vi "ZMQ subscriber example.vi"() -> ()   [LabVIEW 2018]
uses:
  <vilib>/addons/zeromq/socket_type.ctl
  <vilib>/addons/zeromq/socket_options.ctl
  <vilib>/addons/zeromq/zeromq.lvlib
  <vilib>/addons/zeromq/zmq_context.lvclass
  <vilib>/addons/zeromq/zmq_socket.lvclass
panel:
  in  "Display all data":bool
  out "error out":errorcluster
  out "data":string
  out "time between acq":dbl
  in  "Stop":bool
  out "message":string[](array[string])
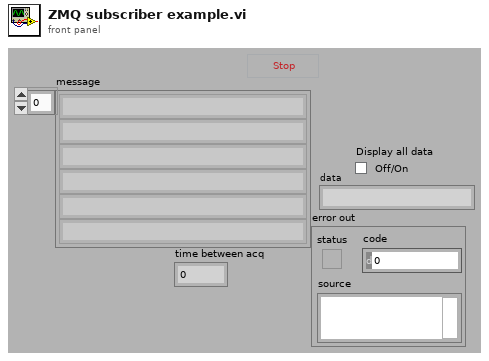
[diagram p1: front panel]
types:
  T1 = typedef "zeromq.lvlib/socket_options.ctl" = enum8{"NONE", "ZMQ_HWM", "<2>", "ZMQ_SWAP", "ZMQ_AFFINITY", "ZMQ_IDENTITY", "ZMQ_SUBSCRIBE", "ZMQ_UNSUBSCRIBE", "ZMQ_RATE", "ZMQ_RECOVERY_IVL", "ZMQ_MCAST_LOOP", "ZMQ_SNDBUF", "ZMQ_RCVBUF", "ZMQ_RCVMORE", "ZMQ_FD", "ZMQ_EVENTS", "ZMQ_TYPE", "ZMQ_LINGER", "ZMQ_RECONNECT_IVL", "ZMQ_BACKLOG", "ZMQ_RECOVERY_IVL_MSEC", "ZMQ_RECONNECT_IVL_MAX", "ZMQ_MAXMSGSIZE", "ZMQ_SNDHWM", "ZMQ_RCVHWM", "ZMQ_MULTICAST_HOPS", "<26>", "ZMQ_RCVTIMEO", "ZMQ_SNDTIMEO", "<29>", "<30>", "ZMQ_IPV4ONLY", "ZMQ_LAST_ENDPOINT", "ZMQ_ROUTER_MANDATORY", "ZMQ_TCP_KEEPALIVE", "ZMQ_TCP_KEEPALIVE_CNT", "ZMQ_TCP_KEEPALIVE_IDLE", "ZMQ_TCP_KEEPALIVE_INTVL", "ZMQ_TCP_ACCEPT_FILTER", "ZMQ_DELAY_ATTACH_ON_CONNECT", "ZMQ_XPUB_VERBOSE"}
  T2 = typedef "zeromq.lvlib/socket_type.ctl" = enum8{"ZMQ_PAIR", "ZMQ_PUB", "ZMQ_SUB", "ZMQ_REQ", "ZMQ_REP", "ZMQ_DEALER", "ZMQ_ROUTER", "ZMQ_PULL", "ZMQ_PUSH", "ZMQ_XPUB", "ZMQ_XSUB"}
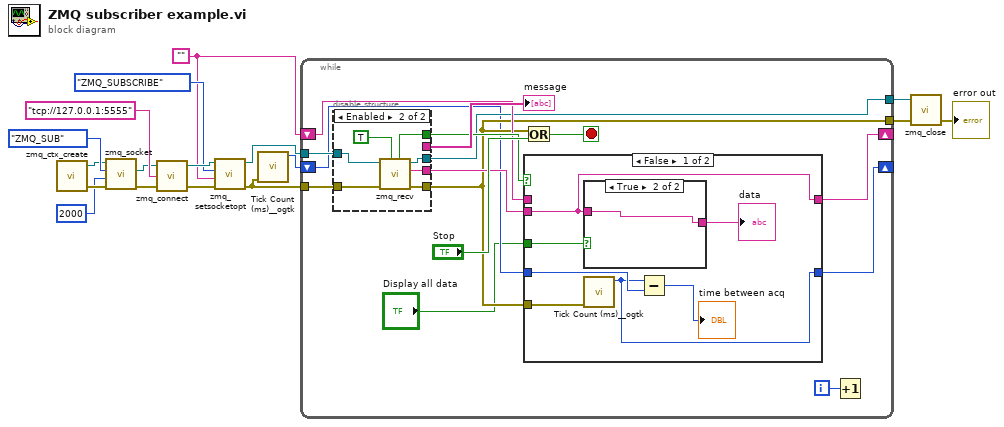
[diagram p0: block diagram]
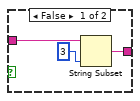
[diagram p2: hidden frame]
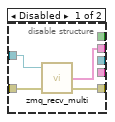
[diagram p4: hidden frame]
diagram:
  w4 = ""
  n1 = call <vilib>:"zmq_ctx_create.vi"() -> ("error out"=w16:errorcluster, "context out"=w8:refnum<class "zmq_context.lvclass">)  [unwired: 4 in]
  n2 = call <vilib>:"zmq_socket.vi"("error in"=w16, "linger (ms)"=2000, "socket type"=socket_type."ZMQ_SUB", "context in"=w8) -> ("error out"=w15:errorcluster, "socket out"=w9:refnum<class "zmq_socket.lvclass">)  [unwired: 1 in, 1 out]
  n3 = call <vilib>:"zmq_connect.vi"("error in"=w15, "endpoint"="tcp://127.0.0.1:5555", "socket in"=w9) -> ("error out"=w13:errorcluster, "socket out"=w14:refnum<class "zmq_socket.lvclass">)  [unwired: 1 in]
  n4 = call <vilib>:"zmq_setsocketopt.vi"("error in"=w13, "value"=w4, "option"=socket_options."ZMQ_SUBSCRIBE", "socket in"=w14) -> ("error out"=w7:errorcluster, "socket out"=w12:refnum<class "zmq_socket.lvclass">)  [unwired: 2 in]
  n5 = call <userlib>:"Tick Count (ms)__ogtk.vi"("error in (no error)"=w7) -> ("millisecond timer value"=w6:u32)  [unwired: 9 in, 1 out]
  n6 = while {
    tunnel: w12 -> [w32]
    tunnel: w7 -> [w30]
    tunnel: [w21] -> w3
    shift-right: [w25] -> _
    shift-left: w4 -> [w23]
    tunnel: [w22] -> w2
    shift-right: [w19] -> _
    shift-left: w6 -> [w20]
    i -> [w27]
    stop <- w28 stop-if-true
    n7 = disable-structure shown="Enabled" {
      disable-tunnel: w32 -> [w49 w56]
      disable-tunnel: [w48 _] -> w31
      disable-tunnel: w30 -> [w47 w55]
      disable-tunnel: [w46 w54] -> w21
      disable-tunnel: [_ w52] -> w26
      disable-tunnel: [_ w51] -> w24
      disable-tunnel: [_ w50] -> w22
      frame Disabled {
        n8 = call <vilib>:"zmq_recv_multi.vi"("error in"=w47, "socket in"=w49) -> ("error out"=w46:errorcluster, "parts"=w48:string[])  [unwired: 1 in, 1 out]
      }
      frame Enabled {
        n9 = call <vilib>:"zmq_recv.vi"("no block? (F)"=TRUE, "error in"=w55, "socket in"=w56) -> ("error out"=w54:errorcluster, "data"=w51:string, "socket out"=w50:refnum<class "zmq_socket.lvclass">, "timeout?"=w52:bool)  [unwired: 2 in, 1 out]
      }
    }
    "message" <- w31
    n10 = Or(x=w21, y="Stop") -> (x .or. y?=w28:bool)
    n11 = case shown="False" w26 {
      tunnel: [w34 w45] -> w25
      tunnel: w24 -> [w34 _]
      tunnel: w23 -> [_ w45]
      tunnel: w21 -> [w39 _]
      tunnel: w20 -> [w38 w44]
      tunnel: [w36 w44] -> w19
      tunnel: "Display all data" -> [w33 _]
      frame False {
        n12 = case shown="True" w33 {
          tunnel: [w42 w43] -> w35
          tunnel: w34 -> [w41 w43]
          frame False {
            n13 = String Subset(string=w41, length (rest)=3 ("length (rest)")) -> (substring=w42:string)  [unwired: 1 in]
          }
          frame True {
          }
        }
        "data" <- w35
        n14 = call <userlib>:"Tick Count (ms)__ogtk.vi"("error in (no error)"=w39) -> ("millisecond timer value"=w36:u32)  [unwired: 9 in, 1 out]
        n15 = Subtract(x=w36, y=w38) -> (x-y=→"time between acq":u32)
      }
      frame True {
      }
    }
    n16 = Increment(x=w27) -> ()  [unwired: 1 out]
  }
  n17 = call <vilib>:"zmq_close.vi"("error in"=w3, "socket"=w2) -> ("error out"=→"error out":errorcluster)  [unwired: 3 in]
